vi "rsscope_core_global.vi"() -> ()   [LabVIEW 2014] (continued)
"Range Table"="RsScope_rngIQInputSampleRate", "Read Callback"="", "Write Callback"="", "Supported Models"="", "Instrument Options"="K11", "Flags"=0, "Help"="Shows the sample rate of capturing the input data in I/Q mode: 20 Gsample/s.\nIf you use R&S RTP134 or R&S RTP164 instruments, you can change the sample rate to 40 Gsample/s.\n\nAvailable Repeated Capabilities:\nNone\n\nRemote-control command(s):\nIQ:INSRate?"}, {"Level"=2, "Class Only"=FALSE, "Identifier"="RSSCOPE_ATTR_IQ_RELATIVE_BANDWIDTH", "Descriptive Name"="IQ Relative Bandwidth", "Data Type"=1, "Command"="IQ:RBW", "Access"=2, "Range Table"="rsscope_rngIQRelativeBandwidth", "Read Callback"="", "Write Callback"="", "Supported Models"="", "Instrument Options"="K11", "Flags"=0, "Help"="Sets the bandwidth factor to define the filter bandwidth.\n\nAvailable Repeated Capabilities:\nNone\n\nRemote-control command(s):\nIQ:RBWidth"}, {"Level"=2, "Class Only"=FALSE, "Identifier"="RSSCOPE_ATTR_IQ_SAMPLE_RATE", "Descriptive Name"="IQ Sample Rate", "Data Type"=1, "Command"="IQ:SRAT", "Access"=2, "Range Table"="rsscope_rngIQSampleRate", "Read Callback"="", "Write Callback"="", "Supported Models"="", "Instrument Options"="K11", "Flags"=0, "Help"="Sets the required sample rate of the output I/Q data.\n\nAvailable Repeated Capabilities:\nNone\n\nRemote-control command(s):\nIQ:SRATe"}, {"Level"=2, "Class Only"=FALSE, "Identifier"="RSSCOPE_ATTR_IQ_RECORD_LENGTH", "Descriptive Name"="IQ Record Length", "Data Type"=0, "Command"="IQ:RLEN", "Access"=2, "Range Table"="rsscope_rngIQRecordLength", "Read Callback"="", "Write Callback"="", "Supported Models"="", "Instrument Options"="K11", "Flags"=0, "Help"="Sets the required record length of the output I/Q data.\n\nAvailable Repeated Capabilities:\nNone\n\nRemote-control command(s):\nIQ:RLENgth"}, {"Level"=2, "Class Only"=FALSE, "Identifier"="RSSCOPE_ATTR_IQ_FILTER_BANDWIDTH", "Descriptive Name"="IQ Filter Bandwidth", "Data Type"=0, "Command"="IQ:BWID?", "Access"=0, "Range Table"="", "Read Callback"="", "Write Callback"="", "Supported Models"="", "Instrument Options"="K11", "Flags"=0, "Help"="Returns the filter bandwidth.\n\nAvailable Repeated Capabilities:\nNone\n\nRemote-control command(s):\nIQ:BWIDth?"}, {"Level"=2, "Class Only"=TRUE, "Identifier"="", "Descriptive Name"="Channel", "Data Type"=0, "Command"="", "Access"=0, "Range Table"="", "Read Callback"="", "Write Callback"="", "Supported Models"="", "Instrument Options"="", "Flags"=0, "Help"="Configures IQ Software properties with Channel repeated capability."}, {"Level"=3, "Class Only"=FALSE, "Identifier"="RSSCOPE_ATTR_IQ_INPUT_TYPE", "Descriptive Name"="IQ Input Type", "Data Type"=0, "Command"="CHAN{Channel}:IQ:INPT", "Access"=2, "Range Table"="rsscope_rngIQInputType", "Read Callback"="", "Write Callback"="", "Supported Models"="", "Instrument Options"="K11", "Flags"=0, "Help"="Sets the type of the input signal.\n\nAvailable Repeated Capabilities:\nChannel: CH1, CH2, CH3, CH4, CHExt\r\n\nRemote-control command(s):\nCHANnel<m>:IQ:INPType"}, {"Level"=3, "Class Only"=FALSE, "Identifier"="RSSCOPE_ATTR_IQ_INPUT_MODE", "Descriptive Name"="IQ Input Mode", "Data Type"=0, "Command"="CHAN{Channel}:IQ:INPM", "Access"=2, "Range Table"="rsscope_rngIQInputMode", "Read Callback"="", "Write Callback"="", "Supported Models"="", "Instrument Options"="K11", "Flags"=0, "Help"="Selects the frequency band of a complex input signal.\n\nAvailable Repeated Capabilities:\nChannel: CH1, CH2, CH3, CH4, CHExt\r\n\nRemote-control command(s):\nCHANnel<m>:IQ:INPMode"}, {"Level"=3, "Class Only"=FALSE, "Identifier"="RSSCOPE_ATTR_IQ_CARRIER_FREQUENCY", "Descriptive Name"="IQ Carrier Frequency", "Data Type"=1, "Command"="CHAN{Channel}:IQ:CFR", "Access"=2, "Range Table"="rsscope_rngIQCarrierFrequency", "Read Callback"="", "Write Callback"="", "Supported Models"="", "Instrument Options"="K11", "Flags"=0, "Help"="Sets the carrier frequency of the modulated RF signal.\n\nAvailable Repeated Capabilities:\nChannel: CH1, CH2, CH3, CH4, CHExt\r\n\nRemote-control command(s):\nCHANnel<m>:IQ:CFRequency"}, {"Level"=3, "Class Only"=FALSE, "Identifier"="RSSCOPE_ATTR_IQ_REAL_SIDEBAND", "Descriptive Name"="IQ Real Sideband", "Data Type"=0, "Command"="CHAN{Channel}:IQ:SBRF", "Access"=2, "Range Table"="rsscope_rngIQRealSideband", "Read Callback"="", "Write Callback"="", "Supported Models"="", "Instrument Options"="K11", "Flags"=0, "Help"="Defines the frequency position of the RF spectrum in the input signal: normal or inverse. The position is important for correct down-conversion and filtering.\n\nAvailable Repeated Capabilities:\nChannel: CH1, CH2, CH3, CH4, CHExt\r\n\nRemote-control command(s):\nCHANnel<m>:IQ:SBRF"}, {"Level"=3, "Class Only"=FALSE, "Identifier"="RSSCOPE_ATTR_IQ_COMPLEX_SIDEBAND", "Descriptive Name"="IQ Complex Sideband", "Data Type"=0, "Command"="CHAN{Channel}:IQ:SBIF", "Access"=2, "Range Table"="rsscope_rngIQComplexSideband", "Read Callback"="", "Write Callback"="", "Supported Models"="", "Instrument Options"="K11", "Flags"=0, "Help"="Defines the sideband and the frequency position of complex modulated input signal in IF range.\n\nAvailable Repeated Capabilities:\nChannel: CH1, CH2, CH3, CH4, CHExt\r\n\nRemote-control command(s):\nCHANnel<m>:IQ:SBIF"}, {"Level"=3, "Class Only"=FALSE, "Identifier"="RSSCOPE_ATTR_IQ_WARNING_ENABLED", "Descriptive Name"="IQ Warning Enabled", "Data Type"=3, "Command"="CHAN{Channel}:IQ:WARN?", "Access"=0, "Range Table"="", "Read Callback"="", "Write Callback"="", "Supported Models"="", "Instrument Options"="K11", "Flags"=0, "Help"="Returns ON if the sampling setup results in an unfavorable combination.\n\nAvailable Repeated Capabilities:\nChannel: CH1, CH2, CH3, CH4, CHExt\r\n\nRemote-control command(s):\nCHANnel<m>:IQ:WARNing[:STATe]?"}, {"Level"=3, "Class Only"=FALSE, "Identifier"="RSSCOPE_ATTR_IQ_WARNING_MESSAGE", "Descriptive Name"="IQ Warning Message", "Data Type"=2, "Command"="CHAN{Channel}:IQ:WARN:MESS?", "Access"=0, "Range Table"="", "Read Callback"="", "Write Callback"="", "Supported Models"="", "Instrument Options"="K11", "Flags"=0, "Help"="Returns the message string if RSSCOPE_ATTR_IQ_WARNING_ENABLED is true.\n\nAvailable Repeated Capabilities:\nChannel: CH1, CH2, CH3, CH4, CHExt\r\n\nRemote-control command(s):\nCHANnel<m>:IQ:WARNing:MESSage?"}, {"Level"=2, "Class Only"=TRUE, "Identifier"="", "Descriptive Name"="Data Output", "Data Type"=0, "Command"="", "Access"=0, "Range Table"="", "Read Callback"="", "Write Callback"="", "Supported Models"="", "Instrument Options"="", "Flags"=0, "Help"="The recorded I/Q data can be extracted using remote control from an external computer."}, {"Level"=1, "Class Only"=TRUE, "Identifier"="", "Descriptive Name"="Spectrum Analysis", "Data Type"=0, "Command"="", "Access"=0, "Range Table"="", "Read Callback"="", "Write Callback"="", "Supported Models"="", "Instrument Options"="", "Flags"=0, "Help"="Contains attributes for Spectrum Analysis."}, {"Level"=2, "Class Only"=FALSE, "Identifier"="RSSCOPE_ATTR_SPECTRUM_ANALYSIS_X_SCALING", "Descriptive Name"="Spectrum Analysis X Scaling", "Data Type"=0, "Command"="CALC:MATH{Math}:FFT:LOGS", "Access"=2, "Range Table"="rsscope_rngEATScale", "Read Callback"="", "Write Callback"="", "Supported Models"="", "Instrument Options"="K18", "Flags"=0, "Help"="Defines the scaling method for the frequency (x-)axis of the spectrogram.\n\nAvailable Repeated Capabilities:\nMath: M1, M2, M3, M4, M5, M6, M7, M8\r\n\nRemote-control command(s):\nCALCulate:MATH<m>:FFT:LOGScale"}, {"Level"=2, "Class Only"=FALSE, "Identifier"="RSSCOPE_ATTR_SPECTRUM_ANALYSIS_WAVEFORM_DATA_SIGNAL_TYPE", "Descriptive Name"="Spectrum Analysis Waveform Data Signal Type", "Data Type"=0, "Command"="CALC:MATH{Math}:DATA:STYP?", "Access"=0, "Range Table"="RsScope_rngDataSignalType", "Read Callback"="", "Write Callback"="", "Supported Models"="", "Instrument Options"="", "Flags"=0, "Help"="Returns the signal type of the source of the math waveform.\n\nAvailable Repeated Capabilities:\nMath: M1, M2, M3, M4, M5, M6, M7, M8\r\n\nRemote-control command(s):\nCALCulate:MATH<m>:DATA:STYPe?"}, {"Level"=2, "Class Only"=FALSE, "Identifier"="RSSCOPE_ATTR_SPECTRUM_ANALYSIS_COLOR_TABLE_MODE", "Descriptive Name"="Spectrum Analysis Color Table Mode", "Data Type"=0, "Command"="CALC:MATH{Math}:FFT:SPEC:CMOD", "Access"=2, "Range Table"="RsScope_rngColorTableMode", "Read Callback"="", "Write Callback"="", "Supported Models"="", "Instrument Options"="", "Flags"=0, "Help"="Selects the color table mode for the frequency analysis display.\n\nAvailable Repeated Capabilities:\nMath: M1, M2, M3, M4, M5, M6, M7, M8\r\n\nRemote-control command(s):\nCALCulate:MATH<m>:FFT:SPECtrogram:CMODe"}, {"Level"=2, "Class Only"=FALSE, "Identifier"="RSSCOPE_ATTR_SPECTRUM_ANALYSIS_USE_COLOR_TABLE", "Descriptive Name"="Spectrum Analysis Use Color Table", "Data Type"=3, "Command"="CALC:MATH{Math}:FFT:USEC", "Access"=2, "Range Table"="", "Read Callback"="", "Write Callback"="", "Supported Models"="", "Instrument Options"="", "Flags"=0, "Help"="If enabled, the selected waveform is displayed according to its assigned color table.\n\nAvailable Repeated Capabilities:\nMath: M1, M2, M3, M4, M5, M6, M7, M8\r\n\nRemote-control command(s):\nCALCulate:MATH<m>:FFT:USEColtab"}, {"Level"=2, "Class Only"=FALSE, "Identifier"="RSSCOPE_ATTR_SPECTRUM_ANALYSIS_SPECTROGRAM_ENABLED", "Descriptive Name"="Spectrum Analysis Spectrogram Enabled", "Data Type"=3, "Command"="CALC:MATH{Math}:FFT:SPEC:STAT", "Access"=2, "Range Table"="", "Read Callback"="", "Write Callback"="", "Supported Models"="", "Instrument Options"="K18", "Flags"=0, "Help"="Enables the spectrogram display for a math waveform.\n\nAvailable Repeated Capabilities:\nMath: M1, M2, M3, M4, M5, M6, M7, M8\r\n\nRemote-control command(s):\nCALCulate:MATH<m>:FFT:SPECtrogram:STATe"}, {"Level"=2, "Class Only"=TRUE, "Identifier"="", "Descriptive Name"="Math2", "Data Type"=0, "Command"="", "Access"=0, "Range Table"="", "Read Callback"="", "Write Callback"="", "Supported Models"="", "Instrument Options"="", "Flags"=0, "Help"="Clas for second math rep_cap."}, {"Level"=3, "Class Only"=FALSE, "Identifier"="RSSCOPE_ATTR_SPECTRUM_ANALYSIS_COUPLED_SPECTRUM", "Descriptive Name"="Spectrum Analysis Coupled Spectrum", "Data Type"=3, "Command"="CALC:MATH{Math}:FFT:COUP:WITH{Math2}", "Access"=2, "Range Table"="", "Read Callback"="", "Write Callback"="", "Supported Models"="", "Instrument Options"="", "Flags"=0, "Help"="Copies the current FFT settings of the selected math waveform (m) to the other selected math waveform (m2), and couples the two waveforms. This can be repeated for all math waveforms.\nIf any FFT setting for any of the coupled spectrums is changed, it is changed for all coupled spectrums.\n\nAvailable Repeated Capabilities:\nMath: M1, M2, M3, M4, M5, M6, M7, M8\r\nMath2: M21, M22, M23, M24, M25, M26, M27, M28\r\n\nRemote-control command(s):\nCALCulate:MATH<m>:FFT:COUPled:WITH<m2>"}, {"Level"=2, "Class Only"=TRUE, "Identifier"="", "Descriptive Name"="Timeline", "Data Type"=0, "Command"="", "Access"=0, "Range Table"="", "Read Callback"="", "Write Callback"="", "Supported Models"="", "Instrument Options"="", "Flags"=0, "Help"="Contains attributes for Spectrum Analysis Timeline."}, {"Level"=3, "Class Only"=FALSE, "Identifier"="RSSCOPE_ATTR_SPECTRUM_ANALYSIS_TIMELINE_ENABLED", "Descriptive Name"="Spectrum Analysis Timeline Enabled", "Data Type"=3, "Command"="CALC:MATH{Math}:FFT:SPEC:TIM{Timeline}:STAT", "Access"=2, "Range Table"="", "Read Callback"="", "Write Callback"="", "Supported Models"="", "Instrument Options"="K18", "Flags"=0, "Help"="Enables one of two possible time lines in a spectrogram diagram. A time line marks a single waveform in the spectrogram, that is: the power vs frequency results for the data acquired at a specific time. After enabling a time line, the results for that time are displayed in the spectrum diagram.\n\nAvailable Repeated Capabilities:\nMath: M1, M2, M3, M4, M5, M6, M7, M8\r\nTimeline: TL1, TL2\r\n\nRemote-control command(s):\nCALCulate:MATH<m>:FFT:SPECtrogram:TIMeline<n>:STATe"}, {"Level"=3, "Class Only"=FALSE, "Identifier"="RSSCOPE_ATTR_SPECTRUM_ANALYSIS_TIMELINE_POSITION", "Descriptive Name"="Spectrum Analysis Timeline Position", "Data Type"=0, "Command"="CALC:MATH{Math}:FFT:SPEC:TIM{Timeline}:POS", "Access"=2, "Range Table"="", "Read Callback"="", "Write Callback"="", "Supported Models"="", "Instrument Options"="K18", "Flags"=0, "Help"="Defines the position of one of the two possible time lines in a spectrogram.\n\nAvailable Repeated Capabilities:\nMath: M1, M2, M3, M4, M5, M6, M7, M8\r\nTimeline: TL1, TL2\r\n\nRemote-control command(s):\nCALCulate:MATH<m>:FFT:SPECtrogram:TIMeline<n>:POSition"}, {"Level"=1, "Class Only"=TRUE, "Identifier"="", "Descriptive Name"="Clock Data Recovery", "Data Type"=0, "Command"="", "Access"=0, "Range Table"="", "Read Callback"="", "Write Callback"="", "Supported Models"="", "Instrument Options"="", "Flags"=0, "Help"="You can define two independent CDR instances to recover clock signals. These clock signals are used for data timing measurements: time interval error, unit interval, and data\nrate (frequency of the clock signal)."}, {"Level"=2, "Class Only"=TRUE, "Identifier"="", "Descriptive Name"="Software", "Data Type"=0, "Command"="", "Access"=0, "Range Table"="", "Read Callback"="", "Write Callback"="", "Supported Models"="", "Instrument Options"="", "Flags"=0, "Help"="Software algorithms that calculate the clock from data signal edges."}, {"Level"=3, "Class Only"=FALSE, "Identifier"="RSSCOPE_ATTR_CDR_SOFTWARE_SERIAL_STANDARD", "Descriptive Name"="CDR Software Serial Standard", "Data Type"=0, "Command"="CDR:SOFT{SW}:SERS", "Access"=2, "Range Table"="RsScope_rngSoftwareSerialStandard", "Read Callback"="", "Write Callback"="", "Supported Models"="", "Instrument Options"="", "Flags"=0, "Help"="Sets the serial standard. The nominal bit rate and bandwidth settings are set according to the selected standard, no estimation is required. Set CUSTOM to adjust the bit rate and the bandwidth manually.\n\nAvailable Repeated Capabilities:\nSW: SW1, SW2\r\n\nRemote-control command(s):\nCDR:SOFTware<m>:SERStandard"}, {"Level"=3, "Class Only"=FALSE, "Identifier"="RSSCOPE_ATTR_CDR_SOFTWARE_BIT_RATE", "Descriptive Name"="CDR Software Bit Rate", "Data Type"=1, "Command"="CDR:SOFT{SW}:BITR", "Access"=2, "Range Table"="rsscope_rngCDRBitRate", "Read Callback"="", "Write Callback"="", "Supported Models"="", "Instrument Options"="", "Flags"=0, "Help"="Sets the quiescent frequency of the PLL. It corresponds to the data rate of the data stream from which the clock is to be recovered.\n\nAvailable Repeated Capabilities:\nSW: SW1, SW2\r\n\nRemote-control command(s):\nCDR:SOFTware<m>:BITRate"}, {"Level"=3, "Class Only"=FALSE, "Identifier"="RSSCOPE_ATTR_CDR_SOFTWARE_BIT_RATE_CORRECTION_ENABLED", "Descriptive Name"="CDR Software Bit Rate Correction Enabled", "Data Type"=3, "Command"="CDR:SOFT{SW}:ESBR:CONT", "Access"=2, "Range Table"="", "Read Callback"="", "Write Callback"="", "Supported Models"="", "Instrument Options"="", "Flags"=0, "Help"="Enables ongoing correction of the bit rate.\n\nAvailable Repeated Capabilities:\nSW: SW1, SW2\r\n\nRemote-control command(s):\nCDR:SOFTware<m>:ESBRate:CONTinuous"}, {"Level"=3, "Class Only"=FALSE, "Identifier"="RSSCOPE_ATTR_CDR_SOFTWARE_BIT_RATE_SOURCE", "Descriptive Name"="CDR Software Bit Rate Source", "Data Type"=0, "Command"="CDR:SOFT{SW}:ESBR:SOUR", "Access"=2, "Range Table"="RsScope_rngBitRateSource", "Read Callback"="", "Write Callback"="", "Supported Models"="", "Instrument Options"="", "Flags"=0, "Help"="Selects the source of the data stream, which is analized to recover the clock.\n\nAvailable Repeated Capabilities:\nSW: SW1, SW2\r\n\nRemote-control command(s):\nCDR:SOFTware<m>:ESBRate:SOURce"}, {"Level"=3, "Class Only"=FALSE, "Identifier"="RSSCOPE_ATTR_CDR_SOFTWARE_ESTIMATE_BIT_RATE_ONCE", "Descriptive Name"="CDR Software Estimate Bit Rate Once", "Data Type"=4, "Command"="CDR:SOFT{SW}:ESBR:BRES", "Access"=1, "Range Table"="", "Read Callback"="", "Write Callback"="", "Supported Models"="", "Instrument Options"="", "Flags"=0, "Help"="Estimates the bit rate once, for the current acquisition.\n\nAvailable Repeated Capabilities:\nSW: SW1, SW2\r\n\nRemote-control command(s):\nCDR:SOFTware<m>:ESBRate:BREStimate"}, {"Level"=3, "Class Only"=FALSE, "Identifier"="RSSCOPE_ATTR_CDR_SOFTWARE_DATA_EDGES", "Descriptive Name"="CDR Software Data Edges", "Data Type"=0, "Command"="CDR:SOFT{SW}:ESL", "Access"=2, "Range Table"="rsscope_rngTriggerSlope", "Read Callback"="", "Write Callback"="", "Supported Models"="", "Instrument Options"="", "Flags"=0, "Help"="Selects the edges of the data stream that are used for the clock recovery.\n\nAvailable Repeated Capabilities:\nSW: SW1, SW2\r\n\nRemote-control command(s):\nCDR:SOFTware<m>:ESLope"}, {"Level"=3, "Class Only"=FALSE, "Identifier"="RSSCOPE_ATTR_CDR_SOFTWARE_INITIAL_PHASE_SYNC", "Descriptive Name"="CDR Software Initial Phase Sync", "Data Type"=0, "Command"="CDR:SOFT{SW}:SYNC", "Access"=2, "Range Table"="rsscope_rngCDRSoftwareInitialPhaseSync", "Read Callback"="", "Write Callback"="", "Supported Models"="", "Instrument Options"="", "Flags"=0, "Help"="Defines the phase reference for the first clock edge.\n\nAvailable Repeated Capabilities:\nSW: SW1, SW2\r\n\nRemote-control command(s):\nCDR:SOFTware<m>:SYNC"}, {"Level"=3, "Class Only"=FALSE, "Identifier"="RSSCOPE_ATTR_CDR_SOFTWARE_SELECTED_RESULTS", "Descriptive Name"="CDR Software Selected Results", "Data Type"=0, "Command"="CDR:SOFT{SW}:RES", "Access"=2, "Range Table"="rsscope_rngCDRSelectedResults", "Read Callback"="", "Write Callback"="", "Supported Models"="", "Instrument Options"="", "Flags"=0, "Help"="Selects measurement to be read.\n\nAvailable Repeated Capabilities:\nSW: SW1, SW2\r\n\nRemote-control command(s):\nCDR:SOFTware<m>:RESults"}, {"Level"=3, "Class Only"=FALSE, "Identifier"="RSSCOPE_ATTR_CDR_SOFTWARE_ALGORITHM", "Descriptive Name"="CDR Software Algorithm", "Data Type"=0, "Command"="CDR:SOFT{SW}:ALG", "Access"=2, "Range Table"="rsscope_rngCDRSoftwareAlgorithm", "Read Callback"="", "Write Callback"="", "Supported Models"="", "Instrument Options"="", "Flags"=0, "Help"="Sets the software algorithm that is used for clock data recovery.\n\nAvailable Repeated Capabilities:\nSW: SW1, SW2\r\n\nRemote-control command(s):\nCDR:SOFTware<m>:ALGorithm"}, {"Level"=3, "Class Only"=FALSE, "Identifier"="RSSCOPE_ATTR_CDR_SOFTWARE_SAMPLING_TIME", "Descriptive Name"="CDR Software Sampling Time", "Data Type"=1, "Command"="CDR:SOFT{SW}:SAMT", "Access"=2, "Range Table"="RsScope_rngCDRSoftwareSamplingTime", "Read Callback"="", "Write Callback"="", "Supported Models"="", "Instrument Options"="", "Flags"=0, "Help"="Sets a sampling time for the clock signal, an offset for the clock edge in relation to the bit start. The clock edge sets the beginning of the unit interval. The sampling time is a number between 0 and 1. Value 0 sets the clock edge to the beginning of the bit period; value 0.5 sets the clock edge to the middle of the bit period.\n\nAvailable Repeated Capabilities:\nSW: SW1, SW2\r\n\nRemote-control command(s):\nCDR:SOFTware<m>:SAMTime"}, {"Level"=3, "Class Only"=FALSE, "Identifier"="RSSCOPE_ATTR_CDR_SOFTWARE_PLL_ORDER", "Descriptive Name"="CDR Software PLL Order", "Data Type"=0, "Command"="CDR:SOFT{SW}:PLL:ORD", "Access"=2, "Range Table"="rsscope_rngCDRPLLOrder", "Read Callback"="", "Write Callback"="", "Supported Models"="", "Instrument Options"="", "Flags"=0, "Help"="Sets the order of the PLL: first or second order. PLL of higher order can compensate for more complex jitter behavior.\n\nAvailable Repeated Capabilities:\nSW: SW1, SW2\r\n\nRemote-control command(s):\nCDR:SOFTware<m>:PLL:ORDer"}, {"Level"=3, "Class Only"=FALSE, "Identifier"="RSSCOPE_ATTR_CDR_SOFTWARE_PLL_DAMPING", "Descriptive Name"="CDR Software PLL Damping", "Data Type"=1, "Command"="CDR:SOFT{SW}:PLL:DAMP", "Access"=2, "Range Table"="rsscope_rngCDRPLLDamping", "Read Callback"="", "Write Callback"="", "Supported Models"="", "Instrument Options"="", "Flags"=0, "Help"="Sets the damping factor, which is only relevant for second order PLL.\n\nAvailable Repeated Capabilities:\nSW: SW1, SW2\r\n\nRemote-control command(s):\nCDR:SOFTware<m>:PLL:DAMPing"}, {"Level"=3, "Class Only"=FALSE, "Identifier"="RSSCOPE_ATTR_CDR_SOFTWARE_PLL_BANDWIDTH", "Descriptive Name"="CDR Software PLL Bandwidth", "Data Type"=1, "Command"="CDR:SOFT{SW}:PLL:BWID", "Access"=2, "Range Table"="", "Read Callback"="", "Write Callback"="", "Supported Models"="", "Instrument Options"="", "Flags"=0, "Help"="Sets the PLL bandwidth. It defines the part of the spectrum that the PLL can follow during synchronization. The PLL bandwidth is usually defined by the transmission standard.\n\nAvailable Repeated Capabilities:\nSW: SW1, SW2\r\n\nRemote-control command(s):\nCDR:SOFTware<m>:PLL:BWIDth"}, {"Level"=3, "Class Only"=FALSE, "Identifier"="RSSCOPE_ATTR_CDR_SOFTWARE_PLL_REL_BANDWIDTH", "Descriptive Name"="CDR Software PLL Relative Bandwidth", "Data Type"=1, "Command"="CDR:SOFT{SW}:PLL:RELB", "Access"=2, "Range Table"="rsscope_rngCDRPLLRelBWSoftware", "Read Callback"="", "Write Callback"="", "Supported Models"="", "Instrument Options"="", "Flags"=0, "Help"="Sets the relative bandwidth, that is the ratio of the nominal bit rate to the PLL bandwidth.\n\nAvailable Repeated Capabilities:\nSW: SW1, SW2\r\n\nRemote-control command(s):\nCDR:SOFTware<m>:PLL:RELBwidth"}, {"Level"=3, "Class Only"=FALSE, "Identifier"="RSSCOPE_ATTR_CDR_SOFTWARE_PLL_REVERSE_LOCK_ENABLED", "Descriptive Name"="CDR Software PLL Reverse Lock Enabled", "Data Type"=3, "Command"="CDR:SOFT{SW}:REVL", "Access"=2, "Range Table"="", "Read Callback"="", "Write Callback"="", "Supported Models"="", "Instrument Options"="", "Flags"=0, "Help"="Enables the reverse lock PLL algorithm. The signal is locked on the first edge.\n\nAvailable Repeated Capabilities:\nSW: SW1, SW2\r\n\nRemote-control command(s):\nCDR:SOFTware<m>:REVLockpll"}, {"Level"=2, "Class Only"=TRUE, "Identifier"="", "Descriptive Name"="Hardware", "Data Type"=0, "Command"="", "Access"=0, "Range Table"="", "Read Callback"="", "Write Callback"="", "Supported Models"="", "Instrument Options"="", "Flags"=0, "Help"="Hhardware Clock Data Recovery (option R&S RTO-K13)."}, {"Level"=3, "Class Only"=FALSE, "Identifier"="RSSCOPE_ATTR_CDR_HARDWARE_SOURCE", "Descriptive Name"="CDR Hardware Source", "Data Type"=0, "Command"="CDR:HARD:SOUR", "Access"=2, "Range Table"="rsscope_rngCDRHardwareSource", "Read Callback"="", "Write Callback"="", "Supported Models"="", "Instrument Options"="K13", "Flags"=0, "Help"="Selects the channel signal that is used for clock recovery.\n\nAvailable Repeated Capabilities:\nNone\n\nRemote-control command(s):\nCDR:HARDware:SOURce"}, {"Level"=3, "Class Only"=FALSE, "Identifier"="RSSCOPE_ATTR_CDR_HARDWARE_SERIAL_STANDARD", "Descriptive Name"="CDR Hardware Serial Standard", "Data Type"=0, "Command"="CDR:HARD:SERS", "Access"=2, "Range Table"="RsScope_rngHardwareSerialStandard", "Read Callback"="", "Write Callback"="", "Supported Models"="", "Instrument Options"="K13", "Flags"=0, "Help"="Sets the serial standard. Set CUSTOM to adjust the bit rate and the bandwidth manually.\n\nAvailable Repeated Capabilities:\nNone\n\nRemote-control command(s):\nCDR:HARDware:SERStandard"}, {"Level"=3, "Class Only"=FALSE, "Identifier"="RSSCOPE_ATTR_CDR_HARDWARE_ESTIMATE_BIT_RATE_ONCE", "Descriptive Name"="CDR Hardware Estimate Bit Rate Once", "Data Type"=4, "Command"="CDR:HARD:BRES", "Access"=1, "Range Table"="", "Read Callback"="", "Write Callback"="", "Supported Models"="", "Instrument Options"="K13", "Flags"=0, "Help"="Estimates the bite rate once, for the current acquisition.\n\nAvailable Repeated Capabilities:\nNone\n\nRemote-control command(s):\nCDR:HARDware:BREStimate"}, {"Level"=3, "Class Only"=FALSE, "Identifier"="RSSCOPE_ATTR_CDR_HARDWARE_BIT_RATE", "Descriptive Name"="CDR Hardware Bit Rate", "Data Type"=1, "Command"="CDR:HARD:BITR", "Access"=2, "Range Table"="", "Read Callback"="", "Write Callback"="", "Supported Models"="", "Instrument Options"="K13", "Flags"=0, "Help"="Sets the quiescent frequency of the PLL. It corresponds to the data rate of the data stream from which the clock is to be recovered.\n\nAvailable Repeated Capabilities:\nNone\n\nRemote-control command(s):\nCDR:HARDware:BITRate"}, {"Level"=3, "Class Only"=FALSE, "Identifier"="RSSCOPE_ATTR_CDR_HARDWARE_DATA_EDGES", "Descriptive Name"="CDR Hardware Data Edges", "Data Type"=0, "Command"="CDR:HARD:ESL", "Access"=2, "Range Table"="rsscope_rngTriggerSlope", "Read Callback"="", "Write Callback"="", "Supported Models"="", "Instrument Options"="K13", "Flags"=0, "Help"="Selects the edges of the data stream that are used for the clock recovery.\n\nAvailable Repeated Capabilities:\nNone\n\nRemote-control command(s):\nCDR:HARDware:ESLope"}, {"Level"=3, "Class Only"=FALSE, "Identifier"="RSSCOPE_ATTR_CDR_HARDWARE_PLL_ORDER", "Descriptive Name"="CDR Hardware PLL Order", "Data Type"=0, "Command"="CDR:HARD:PLL:ORD", "Access"=2, "Range Table"="rsscope_rngCDRPLLOrder", "Read Callback"="", "Write Callback"="", "Supported Models"="", "Instrument Options"="K13", "Flags"=0, "Help"="Sets the order of the PLL: first or second order. PLL of higher order can compensate for more complex jitter behavior.\n\nAvailable Repeated Capabilities:\nNone\n\nRemote-control command(s):\nCDR:HARDware:PLL:ORDer"}, {"Level"=3, "Class Only"=FALSE, "Identifier"="RSSCOPE_ATTR_CDR_HARDWARE_PLL_DAMPING", "Descriptive Name"="CDR Hardware PLL Damping", "Data Type"=1, "Command"="CDR:HARD:PLL:DAMP", "Access"=2, "Range Table"="rsscope_rngCDRPLLDamping", "Read Callback"="", "Write Callback"="", "Supported Models"="", "Instrument Options"="K13", "Flags"=0, "Help"="Sets the damping factor, which is only relevant for second order PLL.\n\nAvailable Repeated Capabilities:\nNone\n\nRemote-control command(s):\nCDR:HARDware:PLL:DAMPing"}, {"Level"=3, "Class Only"=FALSE, "Identifier"="RSSCOPE_ATTR_CDR_HARDWARE_PLL_BANDWIDTH", "Descriptive Name"="CDR Hardware PLL Bandwidth", "Data Type"=1, "Command"="CDR:HARD:PLL:BWID", "Access"=2, "Range Table"="", "Read Callback"="", "Write Callback"="", "Supported Models"="", "Instrument Options"="K13", "Flags"=0, "Help"="Sets the PLL bandwidth. It defines the part of the spectrum that the PLL can follow during synchronization. The PLL bandwidth is usually defined by the transmission standard.\n\nAvailable Repeated Capabilities:\nNone\n\nRemote-control command(s):\nCDR:HARDware:PLL:BWIDth"}, {"Level"=3, "Class Only"=FALSE, "Identifier"="RSSCOPE_ATTR_CDR_HARDWARE_PLL_REL_BANDWIDTH", "Descriptive Name"="CDR Hardware PLL Relative Bandwidth", "Data Type"=0, "Command"="CDR:HARD:PLL:RELB", "Access"=2, "Range Table"="rsscope_rngCDRPLLRelBW", "Read Callback"="", "Write Callback"="", "Supported Models"="", "Instrument Options"="K13", "Flags"=0, "Help"="Sets the relative bandwidth, that is the ratio of the nominal bit rate to the PLL bandwidth.\n\nAvailable Repeated Capabilities:\nNone\n\nRemote-control command(s):\nCDR:HARDware:PLL:RELBwidth"}, {"Level"=3, "Class Only"=FALSE, "Identifier"="RSSCOPE_ATTR_USE_CDR", "Descriptive Name"="Use CDR", "Data Type"=3, "Command"="TRIG:SPAT:CDR", "Access"=2, "Range Table"="", "Read Callback"="", "Write Callback"="", "Supported Models"="", "Instrument Options"="", "Flags"=0, "Help"="Disables the clock source and enables the recovered clock signal generated by hardware CDR.\n\nAvailable Repeated Capabilities:\nNone\n\nRemote-control command(s):\nTRIGger<m>:SPATtern:CDR"}, {"Level"=3, "Class Only"=FALSE, "Identifier"="RSSCOPE_ATTR_CDR_HARDWARE_TRIGGER_UI_OFFSET", "Descriptive Name"="CDR Hardware Trigger UI Offset", "Data Type"=1, "Command"="CDR:HARD:UIOF", "Access"=2, "Range Table"="rsscope_rngCDRTriggerUIOffset", "Read Callback"="", "Write Callback"="", "Supported Models"="", "Instrument Options"="K13", "Flags"=0, "Help"="Defines an offset for the bit start, the beginning of the unit interval. The trigger point corresponds to the clock edge that indicates the bit start. The UI offset is a number between 0 and 1. Value 0 matches sets the clock edge to the beginning of the bit period; value 0.5 sets the clock edge to the middle of the bit period.\n\nAvailable Repeated Capabilities:\nNone\n\nRemote-control command(s):\nCDR:HARDware:UIOFfset"}, {"Level"=1, "Class Only"=TRUE, "Identifier"="", "Descriptive Name"="Display", "Data Type"=0, "Command"="", "Access"=0, "Range Table"="", "Read Callback"="", "Write Callback"="", "Supported Models"="", "Instrument Options"="", "Flags"=0, "Help"="Display settings."}, {"Level"=2, "Class Only"=FALSE, "Identifier"="RSSCOPE_ATTR_DISPLAY_UPDATE", "Descriptive Name"="Display Update", "Data Type"=3, "Command"="SYST:DISP:UPD", "Access"=2, "Range Table"="", "Read Callback"="", "Write Callback"="", "Supported Models"="", "Instrument Options"="", "Flags"=0, "Help"="switches on or off the update of all display elements during remote control.\n\nAvailable Repeated Capabilities:\nNone\n\nRemote-control command(s):\nSYSTem:DISPlay:UPDate"}, {"Level"=2, "Class Only"=FALSE, "Identifier"="RSSCOPE_ATTR_DISPLAY_MESSAGE_ENABLED", "Descriptive Name"="Display Message Enabled", "Data Type"=3, "Command"="SYST:DISP:MESS:STAT", "Access"=2, "Range Table"="", "Read Callback"="", "Write Callback"="", "Supported Models"="", "Instrument Options"="", "Flags"=0, "Help"="Enables and disables the display of an additonal text in remote control.\n\nAvailable Repeated Capabilities:\nNone\n\nRemote-control command(s):\nSYSTem:DISPlay:MESSage:STATe"}, {"Level"=2, "Class Only"=FALSE, "Identifier"="RSSCOPE_ATTR_DISPLAY_MESSAGE_TEXT", "Descriptive Name"="Display Message Text", "Data Type"=2, "Command"="SYST:DISP:MESS", "Access"=2, "Range Table"="", "Read Callback"="", "Write Callback"="", "Supported Models"="", "Instrument Options"="", "Flags"=0, "Help"="Defines an additional text that is displayed during remote control operation.\n\nAvailable Repeated Capabilities:\nNone\n\nRemote-control command(s):\nSYSTem:DISPlay:MESSage[:TEXT]"}, {"Level"=2, "Class Only"=FALSE, "Identifier"="RSSCOPE_ATTR_DISPLAY_GATE_TRANSPARENCY", "Descriptive Name"="Display Gate Transparency", "Data Type"=0, "Command"="DISP:GATE:TRAN", "Access"=2, "Range Table"="RsScope_rngPercentInt", "Read Callback"="", "Write Callback"="", "Supported Models"="", "Instrument Options"="", "Flags"=0, "Help"="Sets the transparency of the area that is defined as measurement or search gate.\n\nAvailable Repeated Capabilities:\nNone\n\nRemote-control command(s):\nDISPlay:GATE:TRANsparency"}, {"Level"=2, "Class Only"=FALSE, "Identifier"="RSSCOPE_ATTR_DISPLAY_CLEAR_RESULTS", "Descriptive Name"="Display Clear Results", "Data Type"=4, "Command"="DISP:CLR", "Access"=1, "Range Table"="", "Read Callback"="", "Write Callback"="", "Supported Models"="", "Instrument Options"="", "Flags"=0, "Help"="Deletes all measurement results including long term measurement and statistics, all waveforms, and the history.\n\nAvailable Repeated Capabilities:\nNone\n\nRemote-control command(s):\nDISPlay:CLR"}, {"Level"=2, "Class Only"=FALSE, "Identifier"="RSSCOPE_ATTR_DISPLAY_RESULTS_ON_EXTERNAL_MONITOR_ENABLED", "Descriptive Name"="Display Results On External Monitor Enabled", "Data Type"=3, "Command"="DISP:EXT:PORD", "Access"=2, "Range Table"="", "Read Callback"="", "Write Callback"="", "Supported Models"="", "Instrument Options"="", "Flags"=0, "Help"="If an external monitor is connected to the instrument, enables the display of result boxes on the external monitor.\n\nAvailable Repeated Capabilities:\nNone\n\nRemote-control command(s):\nDISPlay:EXTended:PORDialogs"}, {"Level"=2, "Class Only"=FALSE, "Identifier"="RSSCOPE_ATTR_DISPLAY_DIALOGS_ON_EXTERNAL_MONITOR_ENABLED", "Descriptive Name"="Display Dialogs On External Monitor Enabled", "Data Type"=3, "Command"="DISP:EXT:POSD", "Access"=2, "Range Table"="", "Read Callback"="", "Write Callback"="", "Supported Models"="", "Instrument Options"="", "Flags"=0, "Help"="If an external monitor is connected to the instrument, enables the display of dialog boxes on the external monitor.\n\nAvailable Repeated Capabilities:\nNone\n\nRemote-control command(s):\nDISPlay:EXTended:POSDialogs"}, {"Level"=2, "Class Only"=TRUE, "Identifier"="", "Descriptive Name"="Signal Colors And Persistence", "Data Type"=0, "Command"="", "Access"=0, "Range Table"="", "Read Callback"="", "Write Callback"="", "Supported Models"="", "Instrument Options"="", "Flags"=0, "Help"="Configures signal colors and persistence settings."}, {"Level"=3, "Class Only"=FALSE, "Identifier"="RSSCOPE_ATTR_PERSISTENCE_STATE", "Descriptive Name"="Persistence State", "Data Type"=3, "Command"="DISP:PERS:STAT", "Access"=2, "Range Table"="", "Read Callback"="", "Write Callback"="", "Supported Models"="", "Instrument Options"="", "Flags"=0, "Help"="If enabled, each new data point in the diagram area remains on the screen for the duration defined using DISPlay:PERSistence:TIME, or as long as DISPlay:PERSistence:INFinite is enabled.\nIf disabled, the signal value is only displayed as long as it actually occurs.\n\nAvailable Repeated Capabilities:\nNone\n\nRemote-control command(s):\nDISPlay:PERSistence[:STATe]"}, {"Level"=3, "Class Only"=FALSE, "Identifier"="RSSCOPE_ATTR_INFINITE_PERSISTENCE", "Descriptive Name"="Infinite Persistence", "Data Type"=3, "Command"="DISP:PERS:INF", "Access"=2, "Range Table"="", "Read Callback"="", "Write Callback"="", "Supported Models"="", "Instrument Options"="", "Flags"=0, "Help"="If persistence is enabled (DISPlay:PERSistence[:STATe]), each new data point in the diagram area remains on the screen infinitely until this command is set to &apos;OFF&apos;.\n\nAvailable Repeated Capabilities:\nNone\n\nRemote-control command(s):\nDISPlay:PERSistence:INFinite"}, {"Level"=3, "Class Only"=FALSE, "Identifier"="RSSCOPE_ATTR_PERSISTENCE_TIME", "Descriptive Name"="Persistence Time", "Data Type"=1, "Command"="DISP:PERS:TIME", "Access"=2, "Range Table"="rsscope_rngPersistenceTime", "Read Callback"="", "Write Callback"="", "Supported Models"="", "Instrument Options"="", "Flags"=0, "Help"="If persistence is enabled (DISPlay:PERSistence[:STATe]), each new data point in the diagram area remains on the screen for the duration defined here.\n\nAvailable Repeated Capabilities:\nNone\n\nRemote-control command(s):\nDISPlay:PERSistence:TIME"}, {"Level"=3, "Class Only"=FALSE, "Identifier"="RSSCOPE_ATTR_PERSISTENCE_RESET", "Descriptive Name"="Persistence Reset", "Data Type"=4, "Command"="DISP:PERS:RES", "Access"=1, "Range Table"="", "Read Callback"="", "Write Callback"="", "Supported Models"="", "Instrument Options"="", "Flags"=0, "Help"="Resets the display, removing persistent values.\n\nAvailable Repeated Capabilities:\nNone\n\nRemote-control command(s):\nDISPlay:PERSistence:RESet"}, {"Level"=3, "Class Only"=FALSE, "Identifier"="RSSCOPE_ATTR_SIGNAL_STYLE_INTENSITY", "Descriptive Name"="Signal Style Intensity", "Data Type"=0, "Command"="DISP:INT", "Access"=2, "Range Table"="rsscope_rngPct", "Read Callback"="", "Write Callback"="", "Supported Models"="", "Instrument Options"="", "Flags"=0, "Help"="This value determines the strength of the waveform line in the diagram. Enter a percentage between 0 (not visible) and 100% (very strong).\nThe exact mapping of the cumulative value occurences according to the assigned color table is guaranteed only if the intensity is set to 50% (default). All other intensity values falsify the mapping but may improve the visibility of the signal.\n\nAvailable Repeated Capabilities:\nNone\n\nRemote-control command(s):\nDISPlay:INTensity"}, {"Level"=3, "Class Only"=FALSE, "Identifier"="RSSCOPE_ATTR_SIGNAL_STYLE", "Descriptive Name"="Signal Style", "Data Type"=0, "Command"="DISP:DIAG:STYL", "Access"=2, "Range Table"="rsscope_rngSignalStyle", "Read Callback"="", "Write Callback"="", "Supported Models"="", "Instrument Options"="", "Flags"=0, "Help"="Select the style in which the waveform is displayed.\n\nAvailable Repeated Capabilities:\nNone\n\nRemote-control command(s):\nDISPlay:DIAGram:STYLe"}, {"Level"=3, "Class Only"=TRUE, "Identifier"="", "Descriptive Name"="Waveform Suffix", "Data Type"=0, "Command"="", "Access"=0, "Range Table"="", "Read Callback"="", "Write Callback"="", "Supported Models"="", "Instrument Options"="", "Flags"=0, "Help"="Selects Waveform Suffix"}, {"Level"=4, "Class Only"=FALSE, "Identifier"="RSSCOPE_ATTR_USE_COLOR_TABLE", "Descriptive Name"="Use Color Table", "Data Type"=3, "Command"="DISP:COL:SIGN{WfmSuffix}:USE", "Access"=2, "Range Table"="", "Read Callback"="", "Write Callback"="", "Supported Models"="", "Instrument Options"="", "Flags"=0, "Help"="If enabled, the selected waveform is displayed according to its assigned color table.\nIf this option is disabled, the default color table is used, i.e. the intensity of the specific signal color varies according to the cumulative occurance of the values.\n\nAvailable Repeated Capabilities:\nWfmSuffix: WfmNone, WfmC1W1, WfmC1W2, WfmC1W3, WfmC2W1, WfmC2W2, WfmC2W3, WfmC3W1, WfmC3W2, WfmC3W3, WfmC4W1, WfmC4W2, WfmC4W3, WfmMath1, WfmMath2, WfmMath3, WfmMath4, WfmRef1, WfmRef2, WfmRef3, WfmRef4, WfmXY1, WfmXY2, WfmXY3, WfmXY4, WfmMeas1, WfmMeas2, WfmMeas3, WfmMeas4, WfmMeas5, WfmMeas6, WfmMeas7, WfmMeas8, WfmSbus1, WfmSbus2, WfmSbus3, WfmSbus4, WfmD0, WfmD1, WfmD2, WfmD3, WfmD4, WfmD5, WfmD6, WfmD7, WfmD8, WfmD9, WfmD10, WfmD11, WfmD12, WfmD13, WfmD14, WfmD15, WfmMSO1, WfmMSO2, WfmMSO3, WfmMSO4, WfmTRK1, WfmTRK2, WfmTRK3, WfmTRK4, WfmTRK5, WfmTRK6, WfmTRK7, WfmTRK8, WfmSpectrum1, WfmSpectrum2, WfmSpectrum3, WfmSpectrum4, WfmSG1TL1, WfmSG1TL2, WfmSG2TL1, WfmSG2TL2, WfmSG3TL1, WfmSG3TL2, WfmSG4TL1, WfmSG4TL2, WfmEye1, WfmEye2, WfmEye3, WfmEye4, WfmZ1V1, WfmZ1V2, WfmZ1V3, WfmZ1V4, WfmZ1I1, WfmZ1I2, WfmZ1I3, WfmZ1I4, WfmZ2V1, WfmZ2V2, WfmZ2V3, WfmZ2V4, WfmZ2I1, WfmZ2I2, WfmZ2I3, WfmZ2I4, WfmDiff1, WfmDiff2, WfmCommon1, WfmCommon2, WfmTDRZ, WfmTDRH, WfmTDRR, WfmMath5, WfmMath6, WfmMath7, WfmMath8, WfmSpectrum5, WfmSpectrum6, WfmSpectrum7, WfmSpectrum8, WfmSG5TL1, WfmSG5TL2, WfmSG6TL1, WfmSG6TL2, WfmSG7TL1, WfmSG7TL2, WfmSG8TL1, WfmSG8TL2, WfmHP1, WfmHP2, WfmHP3, WfmHP4, WfmHP5, WfmHP6, WfmHP7, WfmHP8, WfmHP9, WfmHP10, WfmBathtub1, WfmBathMeas1, WfmStepResp1, WfmSRHist1, WfmSDHist1, WfmTJHist1, WfmDJHist1, WfmDDJHist1, WfmPJHist1, WfmRJOHist1, WfmSRTrack1, WfmTJTrack1, WfmDJTrack1, WfmDDJTrack1, WfmPJTrack1, WfmRJTrack1, WfmTJSpectrum1, WfmDDJSpectrum1, WfmPJSpectrum1, WfmRJSpectrum1, WfmSEye1, WfmBathtub2, WfmBathMeas2, WfmStepResp2, WfmSRHist2, WfmSDHist2, WfmTJHist2, WfmDJHist2, WfmDDJHist2, WfmPJHist2, WfmRJOHist2, WfmSRTrack2, WfmSDTrack2, WfmTJTrack2, WfmDDJTrack2, WfmPJTrack2, WfmRJTrack2, WfmTJSpectrum2, WfmDDJSpectrum2, WfmPJSpectrum2, WfmRJSpectrum2, WfmSEye2, WfmNBathtub1, WfmNBathMeas1, WfmTNHist1, WfmDNHist1, WfmDDNHist1, WfmPNHist1, WfmRNOTrack1, WfmTNTrack1, WfmDDNTrack1, WfmPNTrack1, WfmRNTrack1, WfmTNSpectrum1, WfmDDNSpectrum1, WfmPNSpectrum1, WfmRNSpectrum1, WfmNBathtub2, WfmNBathMeas2, WfmTNHist2, WfmDNHist2, WfmDDNHist2, WfmPNHist2, WfmRNOHist2, WfmTNTrack2, WfmDDNTrack2, WfmPNTrack2, WfmRNTrack2, WfmTNSpectrum2, WfmDDNSpectrum2, WfmPNSpectrum2, WfmRNSpectrum2, WfmPJDHist1, WfmBUJHist1, WfmRJHist1, WfmPJDTrack1, WfmPJDSpectrum1, WfmPJDHist2, WfmBUJHist2, WfmRJHist2, WfmPJDTrack2, WfmPJDSpectrum2, WfmPNDHist1, WfmBUNHist1, WfmRNHist1, WfmPNDTrack1, WfmPNDSpectrum1, WfmPNDHist2, WfmBUNHist2, WfmRNHist2, WfmPNDTrack2, WfmPNDSpectrum2\r\n\nRemote-control command(s):\nDISPlay:COLor:SIGNal<m>:USE"}, {"Level"=4, "Class Only"=FALSE, "Identifier"="RSSCOPE_ATTR_ASSIGN_COLOR_TABLE", "Descriptive Name"="Assign Color Table", "Data Type"=2, "Command"="DISP:COL:SIGN{WfmSuffix}:ASS", "Access"=2, "Range Table"="", "Read Callback"="", "Write Callback"="", "Supported Models"="", "Instrument Options"="", "Flags"=0, "Help"="Adjust the waveform colors to suit your preferences. For each of the following 
